vi "Page_Info_Read.vi"(6 "ctlReferences":T1, 8 "error in (no error)":errorcluster, 11 "AB_WebService in":refnum<class "AB_WebService.lvclass">) -> (0 "error out":errorcluster, 3 "AB_WebService out":refnum<class "AB_WebService.lvclass">)   [LabVIEW 2020, in "AB_WebService.lvclass"]
uses:
  <vilib>/AppBuilder/AB_Classes/WebService/AB_WebService.lvclass
  e:/builds/penguin/labview/branches/2020/dev/dist/vi.lib/AppBuilder/AB_Classes/TargetFile/AB_Targetfile.lvclass
  <resource>/Framework/Providers/Builds/AppBuilder/AB_UI_Page_Info_References.ctl
  <vilib>/AppBuilder/AB_Classes/TargetFile/AB_Targetfile.lvclass
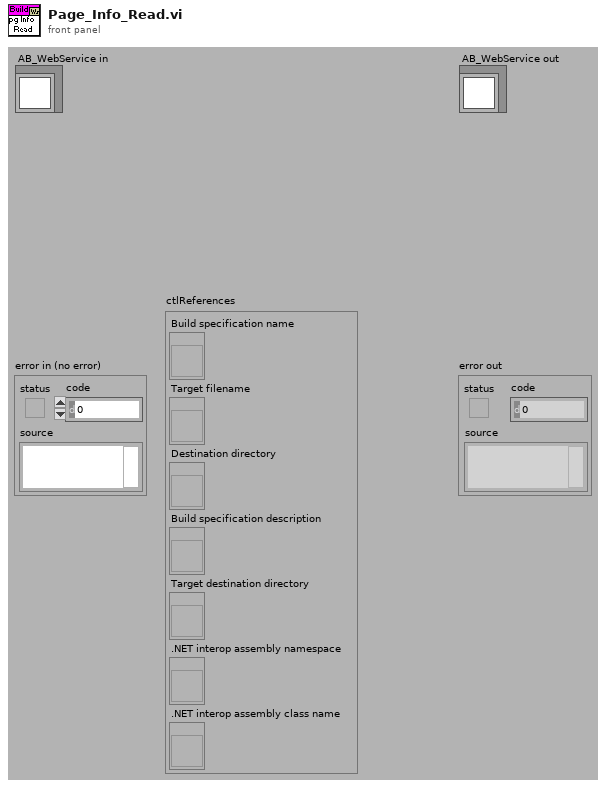
[diagram p1: front panel]
types:
  T1 = typedef "AB_UI_Page_Info_References.ctl" = cluster{"Build specification name":refnum<vi>, "Target filename":refnum<vi>, "Destination directory":refnum<vi>, "Build specification description":refnum<vi>, "Target destination directory":refnum<vi>, ".NET interop assembly namespace":refnum<vi>, ".NET interop assembly class name":refnum<vi>}
  T2 = typedef "AB_Targetfile.ctl" = cluster{"targetfileName":string, "targetfileGUID":string, "enableDebugging":bool, "versionInfo":cluster{"productName":string, "legalCopyright":string, "companyName":string, "internalName":string, "fileDescription":string}, "eng_consolidatedTypeInfo":string, "fastFileFormat":bool, "eng_LEIFBuildData":u32, "versionIndependent":bool}
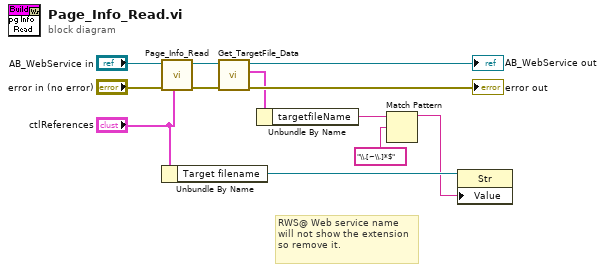
[diagram p0: block diagram]
diagram:
  # "RWS@ Web service name will not show the extension so remove it."
  n1 = call-parent "Page_Info_Read.vi"("ctlReferences"="ctlReferences", "error in (no error)"="error in (no error)", "AB_Targetfile in"="AB_WebService in") -> ("error out"=w6:errorcluster, "AB_Targetfile out"=w8:refnum<class "AB_WebService.lvclass">)  [unwired: 7 in]
  n2 = Unbundle By Name("ctlReferences") -> ("Target filename"=w10:refnum<vi>)
  n3 = call <vilib>:"Get_TargetFile_Data.vi"("error in (no error)"=w6, "AB_Targetfile in"=w8) -> ("error out"=→"error out":errorcluster, "data"=w4:T2, "AB_Targetfile out"=→"AB_WebService out":refnum<class "AB_WebService.lvclass">)  [unwired: 7 in]
  n4 = Unbundle By Name(w4) -> ("targetfileName"=w2:string)
  n5 = Match Pattern(string=w2, regular expression="\\.[~\\.]*$") -> (before substring=w1:string)  [unwired: 4 out]
  n6 = property class="Str"(reference=w10, "Value"=w1) -> ()  [unwired: 1 in, 2 out]
